vi "Global_MCL_piezo.vi"() -> ()   [LabVIEW 2015]
panel:
  out "Autofocus lost":bool
  out "Autofocus stable":bool
  out "Piezo ready":bool
  out "z":dbl
  out "Piezo done":bool
  out "Piezo start":bool
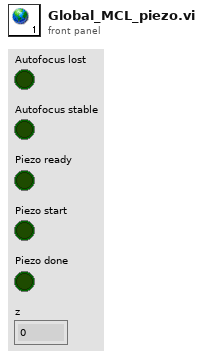
[diagram p1: front panel]
diagram:
